vi "Create.vi"(8 "error in (no error)":errorcluster, 10 "File Paths":path[](array[path])) -> (0 "error out":errorcluster, 3 "LUnit Test Suite V2.lvclass":refnum<class "LUnit Test Suite V2.lvclass">)   [LabVIEW 2020, in "Test Finder V2.lvclass"]
uses:
  Test Finder V2.lvclass
  Test Finder V2.lvclass/Test Finder V2.ctl
  LUnit Test Suite/LUnit Test Suite V2.lvclass
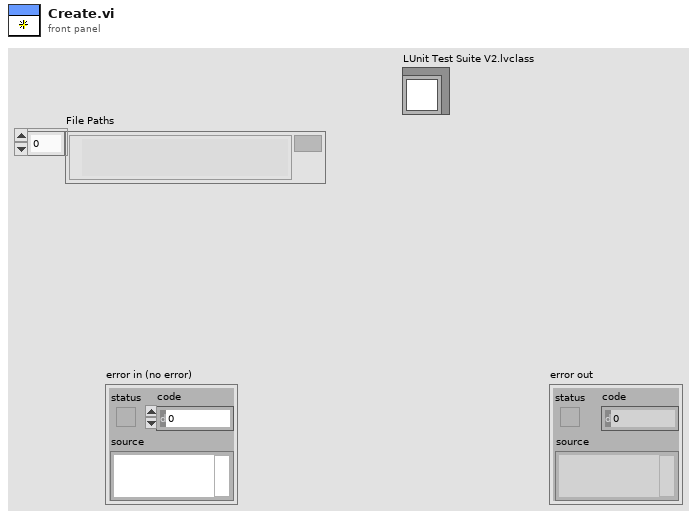
[diagram p1: front panel]
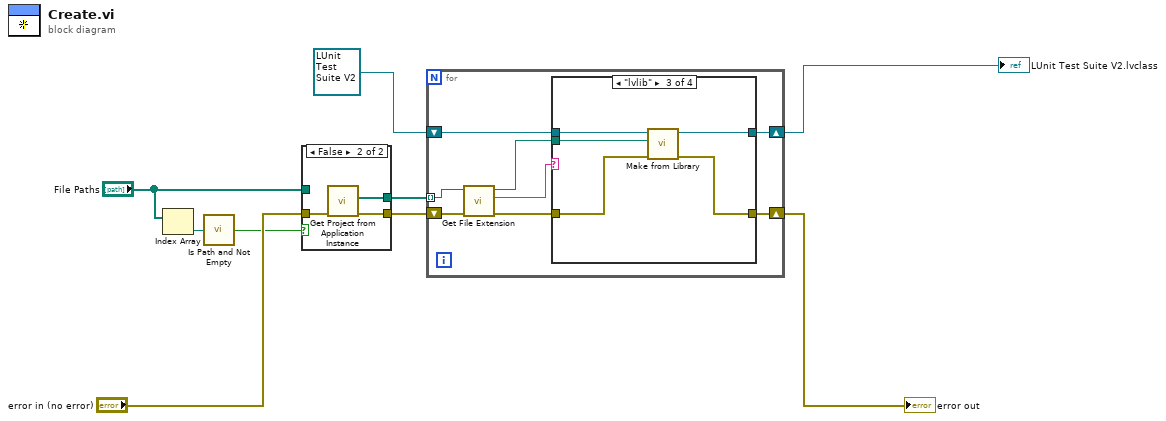
[diagram p0: block diagram]
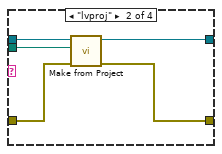
[diagram p3: hidden frame]
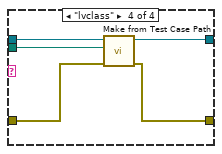
[diagram p4: hidden frame]
diagram:
  n1 = Index Array(array="File Paths") -> (element=w2:path)  [unwired: 1 in]
  n2 = call <vilib>:"Is Path and Not Empty.vi"("path"=w2) -> ("Is Path and Not Empty?"=w1:bool)  [unwired: 4 in]
  n3 = case shown="False" w1 {
    tunnel: "File Paths" -> [w10 _]
    tunnel: "error in (no error)" -> [w11 w13]
    tunnel: [w11 w14] -> w7
    tunnel: [w10 w12] -> w8
    frame True {
    }
    frame False {
      n4 = call "Get Project from Application Instance.vi"("error in (no error)"=w13) -> ("error out"=w14:errorcluster, "Open Projects"=w12:path[])  [unwired: 9 in]
    }
  }
  n5 = for {
    tunnel: w8 -> [w17] mode=indexing
    shift-right: [w19] -> w6
    shift-left: w7 -> [w22]
    shift-right: [w20] -> w4
    shift-left: refnum<class "LUnit Test Suite V2.lvclass"> refnum ("LUnit Test Suite V2.lvclass") -> [w21]
    n6 = call <vilib>:"Get File Extension.vi"("error in (no error)"=w22, "file"=w17) -> ("error out"=w18:errorcluster, "lowercase file extension"=w15:string, "dup file"=w16:path)  [unwired: 5 in, 2 out]
    n7 = case shown="\"lvlib\"" w15 {
      tunnel: w21 -> [w24 w26 w30 w36]
      tunnel: [w24 w25 w31 w35] -> w20
      tunnel: [w23 w29 w34 w39] -> w19
      tunnel: w18 -> [w23 w28 w33 w38]
      tunnel: w16 -> [_ w27 w32 w37]
      frame Default {
      }
      frame "lvproj" {
        n8 = call "Make from Project.vi"("error in (no error)"=w28, "Project Path"=w27, "LUnit Test Suite V2 in"=w26) -> ("error out"=w29:errorcluster, "LUnit Test Suite V2 Out"=w25:refnum<class "LUnit Test Suite V2.lvclass">)  [unwired: 7 in]
      }
      frame "lvlib" {
        n9 = call "Make from Library.vi"("error in (no error)"=w33, "Library Path"=w32, "LUnit Test Suite V2 in"=w30) -> ("error out"=w34:errorcluster, "LUnit Test Suite V2 Out"=w31:refnum<class "LUnit Test Suite V2.lvclass">)  [unwired: 7 in]
      }
      frame "lvclass" {
        n10 = call "Make from Test Case Path.vi"("error in (no error)"=w38, "Test Case"=w37, "LUnit Test Suite V2 in"=w36) -> ("error out"=w39:errorcluster, "LUnit Test Suite V2 out"=w35:refnum<class "LUnit Test Suite V2.lvclass">)  [unwired: 7 in]
      }
    }
  }
  "error out" <- w6
  "LUnit Test Suite V2.lvclass" <- w4
